vi "OracleBusy.vi"(7 "Mode":enum16{"Busy", "Unbusy"}(ring), 8 "Error In":errorcluster) -> (0 "Error Out":errorcluster)   [LabVIEW 2017, in "Server.lvlib" / "Oracle.lvlib"]
doc: "This VI launches OracleBusyDialog.vi which indicates to the user, that the Application is still running properly but he needs to wait for the Oracle DB Query to finish which might take 30-60 seconds. The OracleBusyDialog.vi is aborted after the Oracle Loop is done."
uses:
  Oracle.lvlib
  OracleBusyDialog.vi
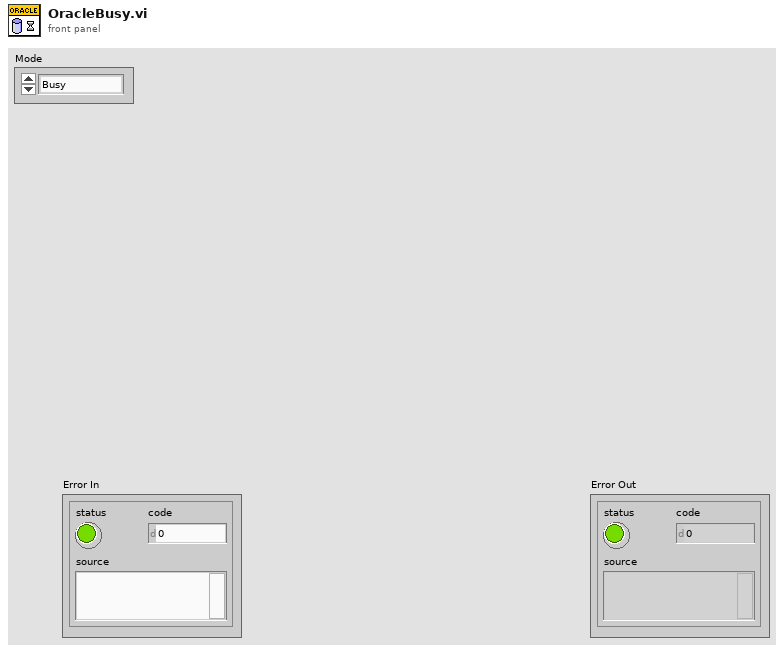
[diagram p1: front panel]
types:
  T1 = enum32{"Invalid", "Standard", "Closed", "Hidden", "Minimized", "Maximized"}
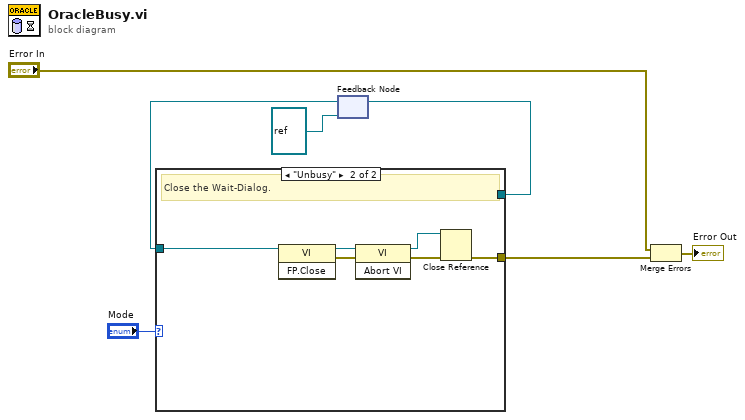
[diagram p0: block diagram]
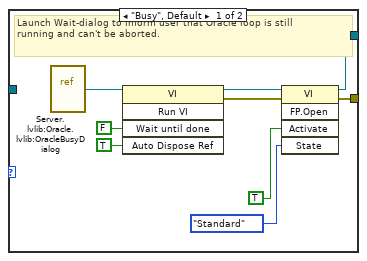
[diagram p2: hidden frame]
diagram:
  n1 = feedback #1(refnum<vi> refnum) -> (w2:refnum<vi>)
  n2 = case shown="\"Unbusy\"" "Mode" {
    tunnel: [w10 _] -> w4
    tunnel: w2 -> [_ w22]
    tunnel: [w12 w19] -> w5
    frame "Busy", Default {
      # "Launch Wait-dialog to inform user that Oracle loop is still\nrunning and can't be aborted."
      n3 = vi-ref "Server.lvlib:Oracle.lvlib:OracleBusyDialog.vi"() -> (w16:refnum<vi>)
      n4 = invoke class="VI" method="Run VI"(reference=w16, "Wait until done"=FALSE ("Wait Until Done"), "Auto Dispose Ref"=TRUE ("Auto Dispose Reference")) -> (reference out=w11:refnum<vi>, error out=w13:errorcluster)  [unwired: 2 in, 3 out]
      n5 = invoke class="VI" method="FP.Open"(reference=w11, error in=w13, "Activate"=TRUE ("Activate?"), "State"=T1."Standard") -> (reference out=w10:refnum<vi>, error out=w12:errorcluster)  [unwired: 1 in, 3 out]
    }
    frame "Unbusy" {
      # "Close the Wait-Dialog."
      n6 = invoke class="VI" method="FP.Close"(reference=w22) -> (reference out=w18:refnum<vi>, error out=w17:errorcluster)  [unwired: 2 in, 1 out]
      n7 = invoke class="VI" method="Abort VI"(reference=w18, error in=w17) -> (reference out=w20:refnum<vi>, error out=w21:errorcluster)  [unwired: 1 in, 1 out]
      n8 = Close Reference(reference=w20, error in (no error)=w21) -> (error out=w19:errorcluster)
    }
  }
  n9 = feedback-in #1(w4) -> ()
  n10 = Merge Errors("Error In", w5) -> (→"Error Out":errorcluster)
